vi "Lidar Motor Controler low features.vi"   [LabVIEW 2009]
uses:
  Test/Lidar Chirp Global.vi
  Motor Control Global.vi
  Motor Output Global.vi
  <vilib>/rvi/FXPMathLib/FxpSinAndCos/XNode/nifxpmath_SinAndCos.xnode
  <vilib>/rvi/FXPMathLib/FxpSinAndCos/subVIs/nifxpmath_SinAndCos_SimConfig.ctl
  <vilib>/rvi/FXPMathLib/FxpSinAndCos/simVIs/DllFxpSinAndCosTemp_sub.vi
  <vilib>/rvi/FXPMathLib/FxpMul/XNode/nifxpmath_Multiplier.xnode
  <vilib>/rvi/FXPMathLib/FxpMul/subVIs/nifxpmath_Mul_SimConfig.ctl
  <vilib>/fxp/LVFixedPointQuantizationPolicyTypeDef.ctl
  <vilib>/fxp/LVFixedPointOverflowPolicyTypeDef.ctl
  <vilib>/rvi/FXPMathLib/FxpMul/simVIs/DllFxpMulTemp_sub.vi
  <vilib>/rvi/FXPMathLib/FxpAdd/XNode/nifxpmath_Add.xnode
  <vilib>/rvi/FXPMathLib/FxpAdd/subVIs/nifxpmath_Add_SimConfig.ctl
  <vilib>/rvi/FXPMathLib/FxpAdd/simVIs/DllFxpAddTemp_sub.vi
  <vilib>/Platform/TimedLoop/XDataNode/XDataNode.xnode
  <vilib>/Platform/TimedLoop/XDataNode/loadlvalarms.vi
  <vilib>/Platform/TimedLoop/XDataNode/timing_clust.ctl
  <vilib>/Platform/TimedLoop/XDataNode/nitl_modes.ctl
  <vilib>/Platform/TimedLoop/XDataNode/wakeup.ctl
  <vilib>/Platform/TimedLoop/XDataNode/XDNodeRunTimeDep.lvlib
types:
  T1 = typedef "Strict Lidar Motor Control Cluster.ctl" = cluster{"Reset Encoder":bool, "Motor Enable":bool, "Motor Voltage":fxp<+/-,20,5>, "Oscillation Frequency (pi rad per 100KHz)":fxp<+/-,20,5>, "Choice of Control Type":enum32{"Direct Voltage Control", "Proportional Control", "PI Control", "Custom Compensator"}, "Choice of Oscillation":enum32{"Oscillate Voltage", "Oscillate Setpoint", "No Oscillation"}, "Choice of Compensation":enum32{"None", "Computed Torque", "Mechanical Advantage", "CT & MA "}, "Gravity Compensation Gain":fxp<+/-,10,1>, "Oscillation Voltage Amplitude":fxp<+/-,20,5>, " Integral Gain":fxp<+/-,20,5>, "Proportional Gain":fxp<+/-,20,5>, "Phi_B Set Point (pi rad)":fxp<+/-,14,4>, "Phi_Lidar - Phi_A":fxp<+/-,10,1>, "Oscillation Setpoint Amplitude":fxp<+/-,14,4>, "Phi_mass-Phi_Lidar":fxp<+/-,10,1>, "Choice of Error":enum32{"Gray Error", "Lidar Error", "Kent Error", "UberKent Error"}, "Phi_A Set Point (pi rad)":fxp<+/-,14,4>, "Phi_Lidar Set Point (pi rad)":fxp<+/-,14,4>, "Phi_B Set Point (enc)":i32, "Phi_B Set Point (pi rad) pre-gain":fxp<+/-,20,5>, "Phi_A Set Point (pi rad) pre-gain":fxp<+/-,20,5>, "Phi_Lidar Set Point (pi rad) pre-gain":fxp<+/-,20,5>, "Phi_B Set Point (enc) pre-gain":fxp<+/-,20,5>, "Lidar Encoder Cap":i32, "Convert (enc) to (pi rad)":fxp<+/-,32,1>}
  T2 = enum32{"Direct Voltage Control", "Proportional Control", "PI Control", "Custom Compensator"}
  T3 = enum32{"Gray Error", "Lidar Error", "Kent Error", "UberKent Error"}
  T4 = typedef "Strict Lidar Motor Indicator Cluster.ctl" = cluster{"Phi_A":fxp<+/-,10,1>, "Phi_B":fxp<+/-,10,1>, "Output Voltage":fxp<+/-,20,5>, "Phi_Lidar":fxp<+/-,10,1>, "Phi_Mass":fxp<+/-,10,1>, "MA":fxp<+/-,8,1>, "Base Output":fxp<+/-,20,5>, "Error":fxp<+/-,20,5>}
  T5 = typedef "XDNodeRunTimeDep.lvlib/timing_clust.ctl" = cluster{"Expected End [f-1]":u64, "Actual End [f-1]":u64, "Finished Late? [f-1]":bool, "Expected End [i-1]":u64, "Actual End [i-1]":u64, "Finished Late? [i-1]":bool, "Expected Start [i]":u64, "Actual Start [i]":u64, "Expected Start [f]":u64, "Actual Start [f]":u64, "Source Name":string, "Structure Name":string, "Period":i64, "Deadline":i64, "Offset":i64, "Start":i64, "Priority":i32, "Timeout":i32, "Mode":T6, "Wakeup Reason":T7, "Error":errorcluster, "Source Type":string, "Secondary Source Type":string, "Global End Time":u64, "Global Start Time":u64, "Frame Duration":u64, "Iteration Duration":u64, "Assigned CPU":i32, "I/O Scan Engine Mode":u32}
  T6 = typedef "XDNodeRunTimeDep.lvlib/nitl_modes.ctl" = enum32{"No Change", "Process missed periods, maintain original phase", "Discard missed periods, maintain original phase", "Process missed periods, ignore original phase", "Discard missed periods, ignore original phase"}
  T7 = typedef "XDNodeRunTimeDep.lvlib/wakeup.ctl" = enum32{"Normal", "Aborted", "Asynchronous wakeup", "Timing source error", "Timed loop error", "Timeout"}
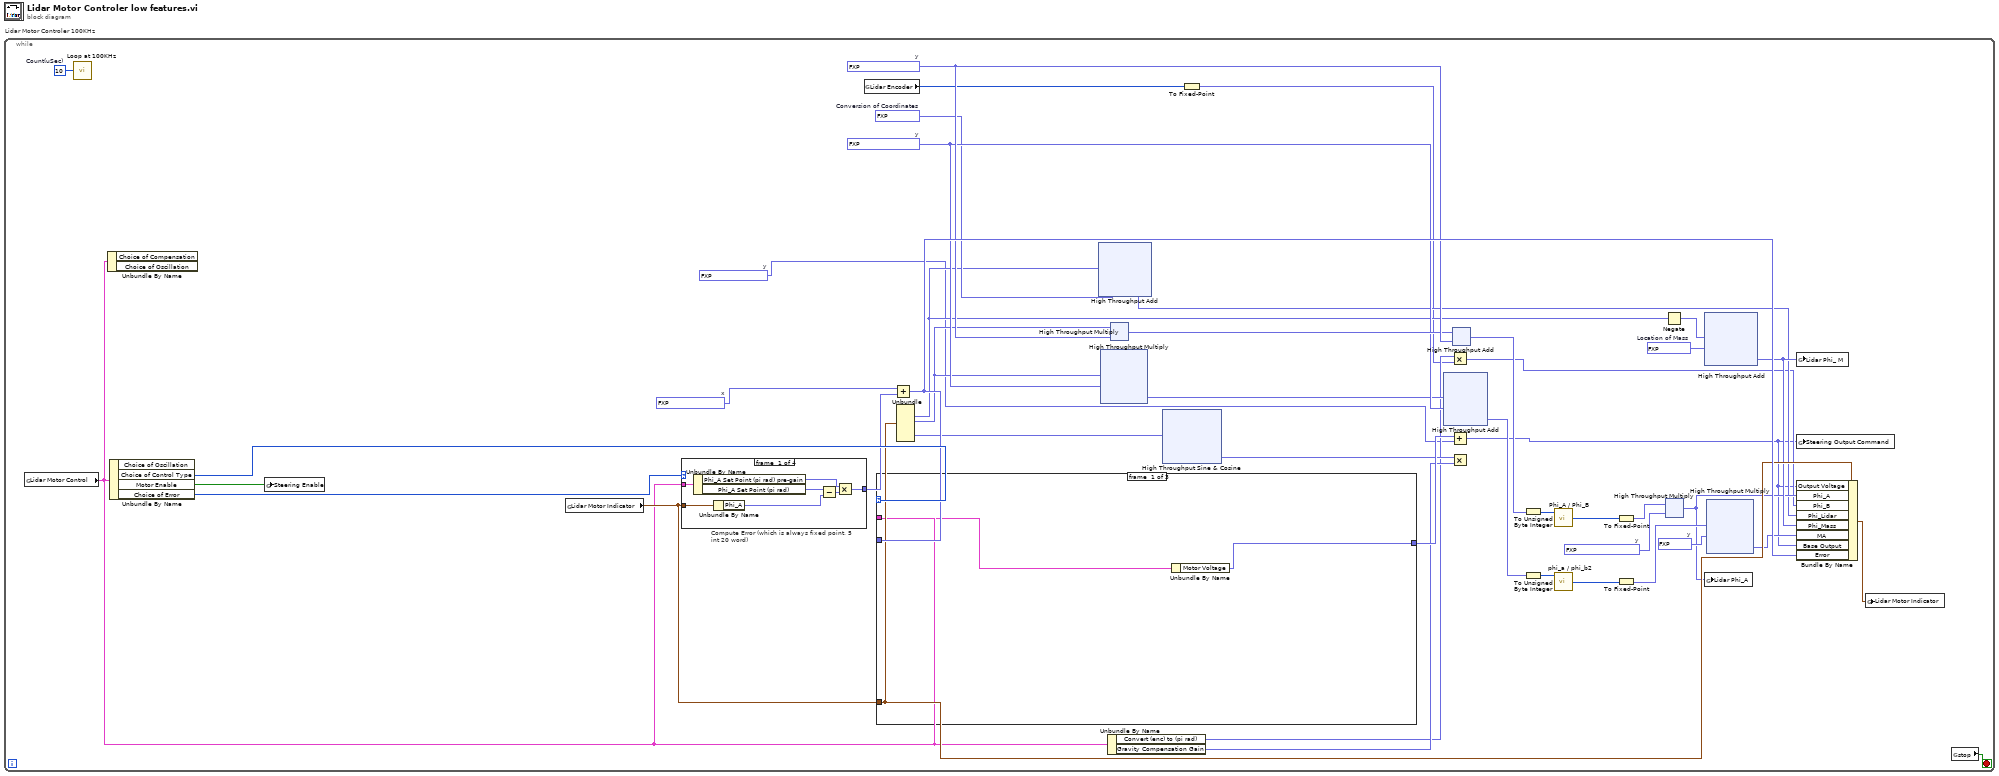
[diagram p0: block diagram]
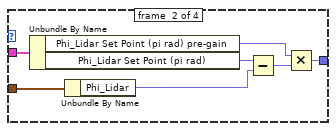
[diagram p2: hidden frame]
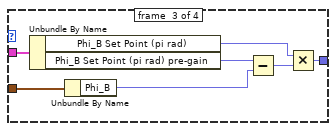
[diagram p3: hidden frame]
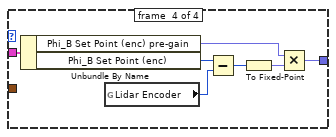
[diagram p4: hidden frame]
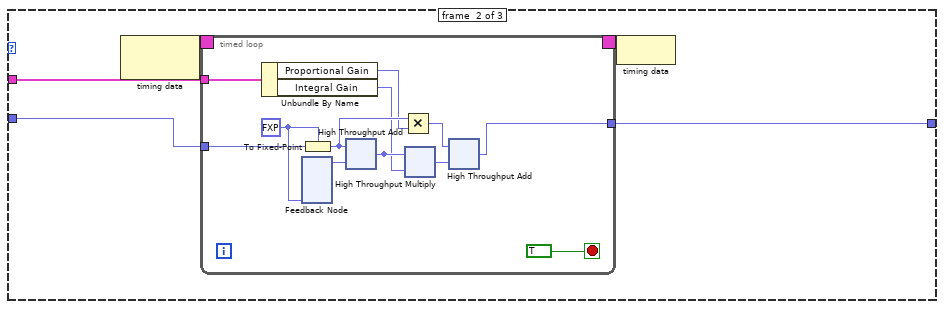
[diagram p5: hidden frame]
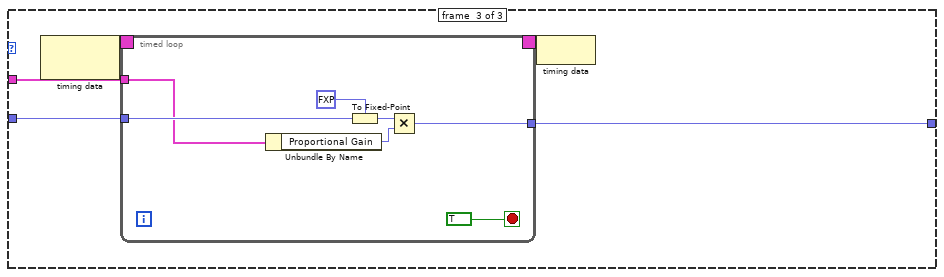
[diagram p6: hidden frame]
diagram:
  n1 = while "Lidar Motor Controler 100KHz" {
    stop <- w44 stop-if-true
    w1 = fxp<+/-,20,5> 0.0  # x
    w3 = fxp<+/-,20,5> 0.0  # y
    w19 = fxp<+/-,10,1> 0.3046875  # Location of Mass
    w21 = fxp<+/-,10,1> 0.103515625  # Conversion of Coordinates
    w26 = fxp<+,8,8> 128.0  # y
    w24 = fxp<+,1,-6> 0.0078125  # y
    w33 = fxp<+,8,8> 128.0  # y
    w31 = fxp<+/-,16,-3> 0.0026035308837890625  # y
    w36 = u32 10  # Count(uSec)
    n2 = global read "Motor Control Global.vi" "Lidar Motor Control"() -> (w7:T1)
    n3 = call "Loop at 100KHz"("Count(uSec)"=w36) -> ()  [unwired: 1 out]
    n4 = Unbundle By Name(w7) -> ()  [unwired: 2 out]
    n5 = Unbundle By Name(w7) -> ("Choice of Control Type"=w43:T2, "Motor Enable"=w42:bool, "Choice of Error"=w40:T3)  [unwired: 1 out]
    n6 = global write "Motor Output Global.vi" "Steering Enable"(w42) -> ()
    n7 = global read "Motor Control Global.vi" "Lidar Motor Indicator"() -> (w18:T4)
    n8 = case "Compute Error (which is always fixed point, 5 int 20 word)" shown="\"Lidar Error\"" w40 {
      tunnel: w7 -> [w297 w308 w310 w319]
      tunnel: w18 -> [w296 w307 w311 _]
      tunnel: [w295 w302 w309 w317] -> w39
      frame #0 {
        n9 = Unbundle By Name(w297) -> ("Phi_A Set Point (pi rad) pre-gain"=w298:fxp<+/-,20,5>, "Phi_A Set Point (pi rad)"=w301:fxp<+/-,14,4>)
        n10 = Unbundle By Name(w296) -> ("Phi_A"=w300:fxp<+/-,10,1>)
        n11 = Subtract(x=w301, y=w300) -> (x-y=w299:fxp<+/-,20,5>)
        n12 = Multiply(x=w298, y=w299) -> (x*y=w295:fxp<+/-,20,5>)
      }
      frame #1 {
        n13 = Unbundle By Name(w308) -> ("Phi_Lidar Set Point (pi rad) pre-gain"=w303:fxp<+/-,20,5>, "Phi_Lidar Set Point (pi rad)"=w306:fxp<+/-,14,4>)
        n14 = Unbundle By Name(w307) -> ("Phi_Lidar"=w305:fxp<+/-,10,1>)
        n15 = Subtract(x=w306, y=w305) -> (x-y=w304:fxp<+/-,20,5>)
        n16 = Multiply(x=w303, y=w304) -> (x*y=w302:fxp<+/-,20,5>)
      }
      frame #2 {
        n17 = Unbundle By Name(w310) -> ("Phi_B Set Point (pi rad)"=w312:fxp<+/-,14,4>, "Phi_B Set Point (pi rad) pre-gain"=w315:fxp<+/-,20,5>)
        n18 = Unbundle By Name(w311) -> ("Phi_B"=w314:fxp<+/-,10,1>)
        n19 = Subtract(x=w315, y=w314) -> (x-y=w313:fxp<+/-,20,5>)
        n20 = Multiply(x=w312, y=w313) -> (x*y=w309:fxp<+/-,20,5>)
      }
      frame #3 {
        n21 = Unbundle By Name(w319) -> ("Phi_B Set Point (enc) pre-gain"=w320:fxp<+/-,20,5>, "Phi_B Set Point (enc)"=w322:i32)
        n22 = global read "Motor Control Global.vi" "Lidar Encoder"() -> (w318:i32)
        n23 = Subtract(x=w322, y=w318) -> (x-y=w321:i32)
        n24 = To Fixed-Point(number=w321) -> (fixed-point=w316:fxp<+/-,32,32>)  [unwired: 1 in]
        n25 = Multiply(x=w320, y=w316) -> (x*y=w317:fxp<+/-,20,5>)
      }
    }
    n26 = global read "Motor Control Global.vi" "Lidar Encoder"() -> (w8:i32)
    n27 = Add(x=w1, y=w39) -> (x+y=w37:fxp<+/-,20,5>)
    n28 = case shown="\"Direct Voltage Control\", Default" w43 {
      tunnel: [w323 w328 w432] -> w38
      tunnel: w37 -> [_ w329 w431]
      tunnel: w7 -> [w324 w327 w430]
      tunnel: w18 -> [_ _ _]
      frame #0 {
        n29 = Unbundle By Name(w324) -> ("Motor Voltage"=w323:fxp<+/-,20,5>)
      }
      frame #1 {
        n30 = node-c288() -> (w326:T5)  [unwired: 1 in]
        n31 = timed-loop {
          timing: w326 -> [_]
          timing-out: [_] -> w325
          tunnel: w329 -> [w335]
          tunnel: [w334] -> w328
          tunnel: w327 -> [w333]
          stop <- TRUE stop-if-true
          w339 = fxp<+/-,20,5> 0.0 ("fixed-point type")
          n32 = Unbundle By Name(w333) -> ("Proportional Gain"=w332:fxp<+/-,20,5>, "Integral Gain"=w331:fxp<+/-,20,5>)
          n33 = feedback #1(w339) -> (w338:fxp<+/-,20,5>)
          n34 = To Fixed-Point(fixed-point type=w339, number=w335) -> (fixed-point=w337:fxp<+/-,20,5>)
          n35 = xnode "High Throughput Add"("x"=w337, "y"=w338) -> ("x+y"=w340:fxp<+/-,20,5>)
          n36 = Multiply(x=w337, y=w332) -> (x*y=w336:fxp<+/-,20,5>)
          n37 = xnode "High Throughput Multiply"("x"=w340, "y"=w331) -> ("x*y"=w341:fxp<+/-,20,5>)
          n38 = xnode "High Throughput Add"("x"=w336, "y"=w341) -> ("x+y"=w334:fxp<+/-,20,5>)
        }
        n39 = node-c288(w325) -> ()
      }
      frame #2 {
        n40 = node-c288() -> (w429:T5)  [unwired: 1 in]
        n41 = timed-loop {
          timing: w429 -> [_]
          timing-out: [_] -> w428
          tunnel: [w437] -> w432
          tunnel: w431 -> [w436]
          tunnel: w430 -> [w435]
          stop <- TRUE stop-if-true
          n42 = Unbundle By Name(w435) -> ("Proportional Gain"=w434:fxp<+/-,20,5>)
          n43 = To Fixed-Point(fixed-point type=fxp<+/-,20,5> 0.0, number=w436) -> (fixed-point=w438:fxp<+/-,20,5>)
          n44 = Multiply(x=w438, y=w434) -> (x*y=w437:fxp<+/-,20,5>)
        }
        n45 = node-c288(w428) -> ()
      }
    }
    n46 = Unbundle(w18) -> ("Output Voltage"=w15:fxp<+/-,20,5>, "Phi_Lidar"=w16:fxp<+/-,10,1>, "Base Output"=w13:fxp<+/-,20,5>)  [unwired: 5 out]
    n47 = xnode "High Throughput Add"("x"=w15, "y"=w21) -> ("x+y"=w11:fxp<+/-,10,1>)
    n48 = xnode "High Throughput Multiply"("x"=w16, "y"=w26) -> ("x*y"=w25:fxp<+/-,8,8>)
    n49 = Unbundle By Name(w7) -> ("Convert (enc) to (pi rad)"=w5:fxp<+/-,32,1>, "Gravity Compensation Gain"=w9:fxp<+/-,10,1>)
    n50 = xnode "High Throughput Multiply"("x"=w16, "y"=w33) -> ("x*y"=w32:fxp<+/-,8,8>)
    n51 = xnode "High Throughput Sine & Cosine"("x (pi)"=w13) -> ("cos(x)"=w10:fxp<+/-,16,2>)  [unwired: 1 out]
    n52 = To Fixed-Point(number=w8) -> (fixed-point=w4:fxp<+/-,32,32>)  [unwired: 1 in]
    n53 = xnode "High Throughput Add"("x"=w25, "y"=w26) -> ("x+y"=w27:fxp<+,8,8>)
    n54 = Multiply(x=w5, y=w4) -> (x*y=w6:fxp<+/-,10,1>)
    n55 = Add(x=w38, y=w3) -> (x+y=w2:fxp<+/-,20,5>)
    n56 = Multiply(x=w10, y=w9) -> ()  [unwired: 1 out]
    n57 = xnode "High Throughput Add"("x"=w32, "y"=w33) -> ("x+y"=w34:fxp<+,8,8>)
    n58 = To Unsigned Byte Integer(number=w34) -> (unsigned 8bit integer=w35:u8)
    n59 = To Unsigned Byte Integer(number=w27) -> (unsigned 8bit integer=w28:u8)
    n60 = call "Phi_A / Phi_B"("address"=w35) -> ("data out"=w29:i8)  [unwired: 8 in]
    n61 = call "phi_a / phi_b2"("address"=w28) -> ("data out"=w22:i8)  [unwired: 8 in]
    n62 = To Fixed-Point(number=w29) -> (fixed-point=w30:fxp<+/-,8,8>)  [unwired: 1 in]
    n63 = To Fixed-Point(number=w22) -> (fixed-point=w23:fxp<+/-,8,8>)  [unwired: 1 in]
    n64 = Negate(x=w15) -> (-x=w20:fxp<+/-,21,6>)
    n65 = xnode "High Throughput Multiply"("x"=w30, "y"=w31) -> ("x*y"=w12:fxp<+/-,10,1>)
    n66 = xnode "High Throughput Add"("x"=w20, "y"=w19) -> ("x+y"=w14:fxp<+/-,10,1>)
    n67 = global write "Lidar Chirp Global.vi" "Lidar Phi_A"(w12) -> ()
    n68 = xnode "High Throughput Multiply"("x"=w23, "y"=w24) -> ("x*y"=w17:fxp<+/-,8,1>)
    n69 = global write "Lidar Chirp Global.vi" "Lidar Phi_ M"(w14) -> ()
    n70 = global write "Motor Output Global.vi" "Steering Output Command"(w2) -> ()
    n71 = Bundle By Name(cluster=w18, "Output Voltage"=w2, "Phi_A"=w12, "Phi_B"=w6, "Phi_Lidar"=w11, "Phi_Mass"=w14, "MA"=w17, "Base Output"=w2, "Error"=w37) -> (w41:T4)
    n72 = global write "Motor Control Global.vi" "Lidar Motor Indicator"(w41) -> ()
    n73 = global read "Motor Control Global.vi" "stop"() -> (w44:bool)
  }
